vi "configureFunction.vi"(8 "error in (no error)":errorcluster, 9 "Config":i32, 10 "Function":i32, 11 "Mockbus in":refnum<class "Mockbus.lvclass">) -> (0 "error out":errorcluster, 3 "Mockbus out":refnum<class "Mockbus.lvclass">)   [LabVIEW 2015, in "RTMockbus.lvlib" / "Mockbus.lvclass"]
uses:
  Mockbus.lvclass
  Mockbus.lvclass/Mockbus.ctl
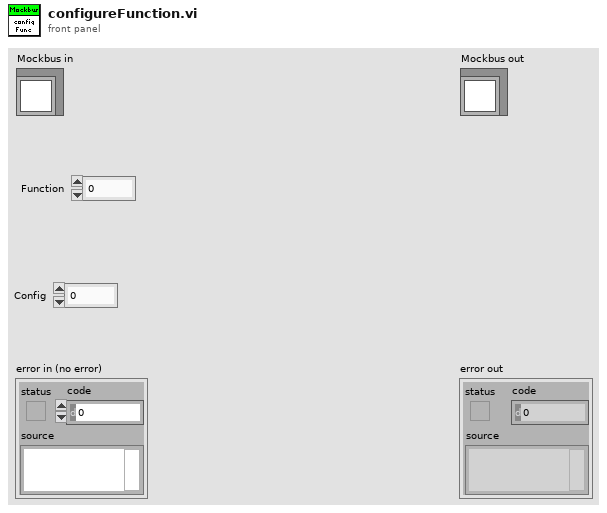
[diagram p1: front panel]
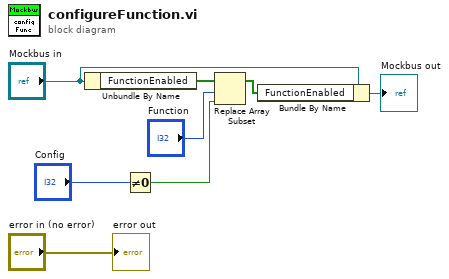
[diagram p0: block diagram]
diagram:
  n1 = Unbundle By Name("Mockbus in") -> ("FunctionEnabled"=w6:bool[])
  n2 = Not Equal To 0?(x="Config") -> (x != 0?=w3:bool)
  n3 = Replace Array Subset(array=w6, new element=w3, index="Function") -> (w2:bool[])
  n4 = Bundle By Name(cluster="Mockbus in", "FunctionEnabled"=w2) -> (→"Mockbus out":refnum<class "Mockbus.lvclass">)
  "error out" <- "error in (no error)"
